vi "OnDataDrag3.vi"(0 "XRef":T20, 1 "Point":T18, 2 "String":T12, 3 "Path":T17, 4 "ProjectItemRefs":T15, 5 "GObjRefs":T13, 6 "State In":T1) -> (14 "Reply":T11, 15 "Fatal Error Out":T10, 16 "State Out":T1)   [LabVIEW 2020, in "FlexBlock.xnode"]
uses:
  FlexBlock.xnode
  <vilib>/XNodeSupport/XNodeXNodeRef.ctl
  <vilib>/XNodeSupport/XNodePoint.ctl
  <vilib>/XNodeSupport/XNodeInt.ctl
  <vilib>/XNodeSupport/XNodeString.ctl
  <vilib>/XNodeSupport/XNodePath.ctl
  <vilib>/XNodeSupport/XNodeProjItemRefArray.ctl
  <vilib>/XNodeSupport/XNodeProjItemRef.ctl
  <vilib>/XNodeSupport/XNodeGObjRefArray.ctl
  <vilib>/XNodeSupport/XNodeGObjRef.ctl
  State.ctl
  FlexBlocks/Type Descriptor.ctl
  FlexBlocks/Terminal Direction.ctl
  FlexBlocks/Value Mode.ctl
  FlexBlocks/Terminal State.ctl
  FlexBlocks/Special Terminal.ctl
  FlexBlocks/Errors.ctl
  <vilib>/picture/picture.llb/imagedata.ctl
  FlexBlocks/Calculated Sizes.ctl
  <vilib>/XNodeSupport/XNodeStringArray.ctl
  <vilib>/XNodeSupport/XNodeErrorCluster.ctl
  <vilib>/XNodeSupport/NI_XNodeSupport.lvlib
  FlexBlocks/FlexBlocks.lvlib
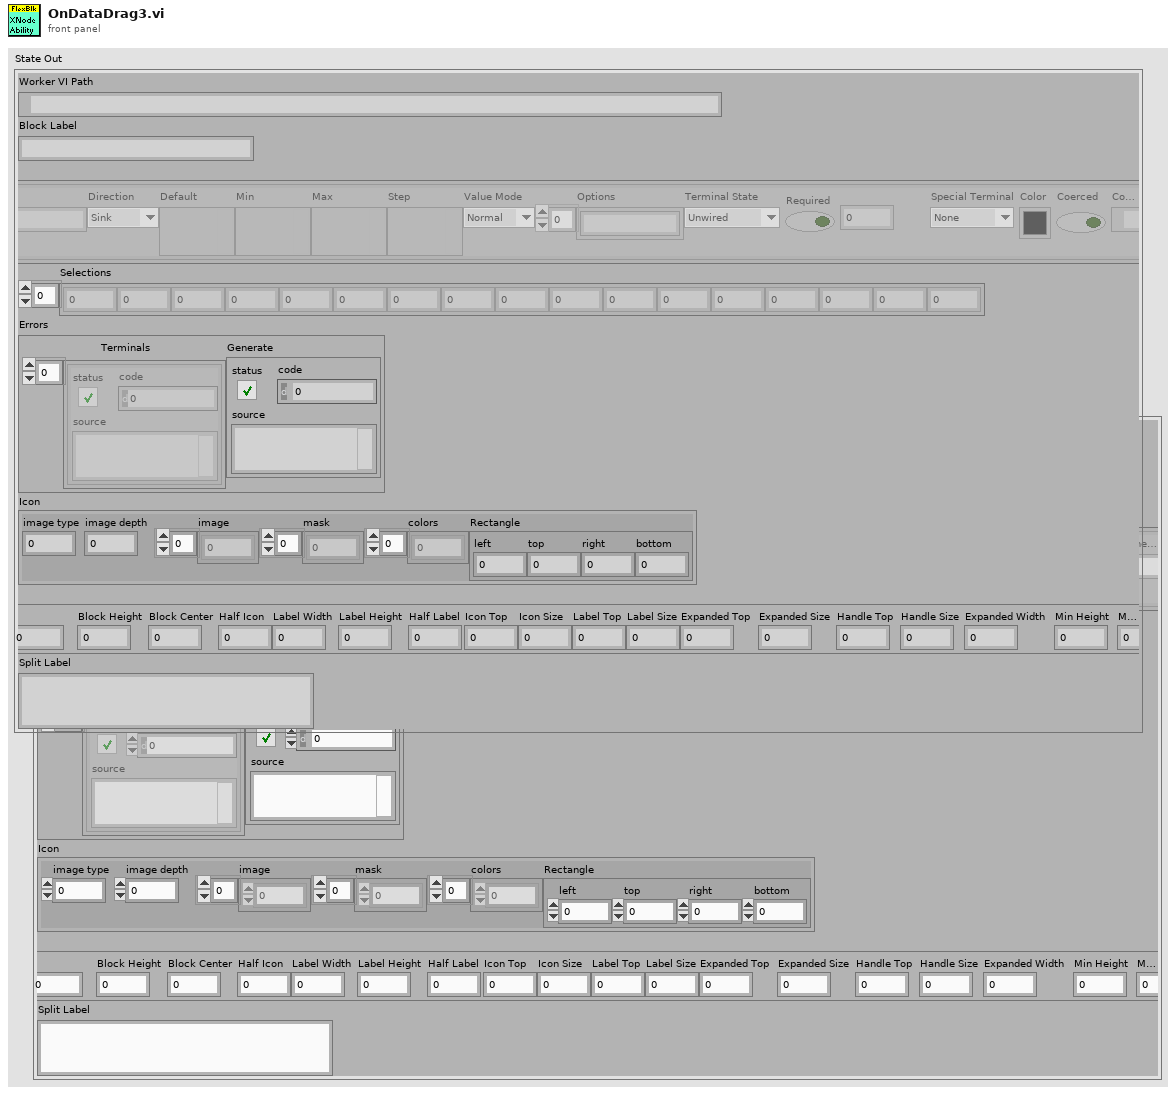
[diagram p1: front panel]
types:
  T1 = typedef "FlexBlock.xnode/State.ctl" = cluster{"Worker VI Path":path, "Block Label":string, "Types":T2[], "Selections":i32[], "Errors":T7, "Icon":T8, "Calcd Sizes":T9, "Split Label":string}
  T2 = typedef "FlexBlocks.lvlib/Type Descriptor.ctl" = cluster{"Name":string, "Direction":T3, "Default":variant, "Min":variant, "Max":variant, "Step":variant, "Value Mode":T4, "Options":string[], "Terminal State":T5, "Required":bool, "Connpane Index":i32, "Special Terminal":T6, "Color":u32, "Coerced":bool, "Connection Path":path}
  T3 = typedef "FlexBlocks.lvlib/Terminal Direction.ctl" = enum16{"Sink", "Source"}
  T4 = typedef "FlexBlocks.lvlib/Value Mode.ctl" = enum16{"Normal", "Range", "Select"}
  T5 = typedef "FlexBlocks.lvlib/Terminal State.ctl" = enum16{"Unwired", "BadType", "BadRef", "Channel", "Value", "Control Ref"}
  T6 = typedef "FlexBlocks.lvlib/Special Terminal.ctl" = enum16{"None", "Action", "Init", "Tag", "State in", "State out", "Error"}
  T7 = typedef "FlexBlocks.lvlib/Errors.ctl" = cluster{"Terminals":errorcluster[], "Generate":errorcluster}
  T8 = typedef "imagedata.ctl" = cluster{"image type":i32, "image depth":i32, "image":u8[], "mask":u8[], "colors":u32[], "Rectangle":cluster{"left":i16, "top":i16, "right":i16, "bottom":i16}}
  T9 = typedef "FlexBlocks.lvlib/Calculated Sizes.ctl" = cluster{"Text Width":i32, "Text Height":i32, "Half Text":i32, "Block Width":i32, "Block Height":i32, "Block Center":i32, "Half Icon":i32, "Label Width":i32, "Label Height":i32, "Half Label":i32, "Icon Top":i32, "Icon Size":i32, "Label Top":i32, "Label Size":i32, "Expanded Top":i32, "Expanded Size":i32, "Handle Top":i32, "Handle Size":i32, "Expanded Width":i32, "Min Height":i32, "Max Height":i32}
  T10 = typedef "NI_XNodeSupport.lvlib/XNodeErrorCluster.ctl" = errorcluster
  T11 = typedef "NI_XNodeSupport.lvlib/XNodeStringArray.ctl" = T12[]
  T12 = typedef "NI_XNodeSupport.lvlib/XNodeString.ctl" = string
  T13 = typedef "NI_XNodeSupport.lvlib/XNodeGObjRefArray.ctl" = T14[]
  T14 = typedef "NI_XNodeSupport.lvlib/XNodeGObjRef.ctl" = refnum<vi>
  T15 = typedef "NI_XNodeSupport.lvlib/XNodeProjItemRefArray.ctl" = T16[]
  T16 = typedef "NI_XNodeSupport.lvlib/XNodeProjItemRef.ctl" = refnum<vi>
  T17 = typedef "NI_XNodeSupport.lvlib/XNodePath.ctl" = path
  T18 = typedef "NI_XNodeSupport.lvlib/XNodePoint.ctl" = cluster{"H":T19, "V":T19}
  T19 = typedef "NI_XNodeSupport.lvlib/XNodeInt.ctl" = i32
  T20 = typedef "NI_XNodeSupport.lvlib/XNodeXNodeRef.ctl" = refnum<vi>
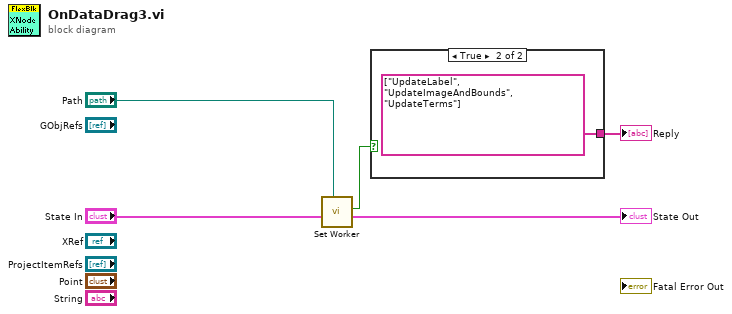
[diagram p0: block diagram]
diagram:
  n1 = call "Set Worker.vi"("Worker VI Path"="Path", "State In"="State In") -> ("State"=→"State Out":T1, "Is Worker?"=w1:bool)  [unwired: 8 in]
  n2 = case shown="True" w1 {
    tunnel: [_ T11 ["UpdateLabel", "UpdateImageAndBounds", "UpdateTerms"] ("Reply")] -> w2
    frame False {
    }
    frame True {
    }
  }
  "Reply" <- w2
